vi "VI Tree.vi"   [LabVIEW 2015, in "Keithley 2600 Series.lvlib"]
doc: "This is the instrument driver for the Keithley 2600 Series. The VI Tree displays all the user-callable VIs of the instrument driver in an organized table."
uses:
  Keithley 2600 Series.lvlib
  Configure/Factory Script/Configure Tag Current Pulse (Linear).vi
  Configure/Factory Script/Configure Tag Voltage Pulse (Linear).vi
  Configure/Source/Configure Source (Level).vi
  Data/Read Asynchronous Measurement (Current).vi
  Data/Read Current (Linear Voltage Sweep).vi
  Data/Read Measurement (Current).vi
  Data/Read Transconductance (Current).vi
  Data/Read Voltage (Linear Current Sweep).vi
panel:
  # "(c) 2020 - 2022 National Instruments.  ALL RIGHTS RESERVED."
  # "SEE DIAGRAM\nFOR VI TREE."
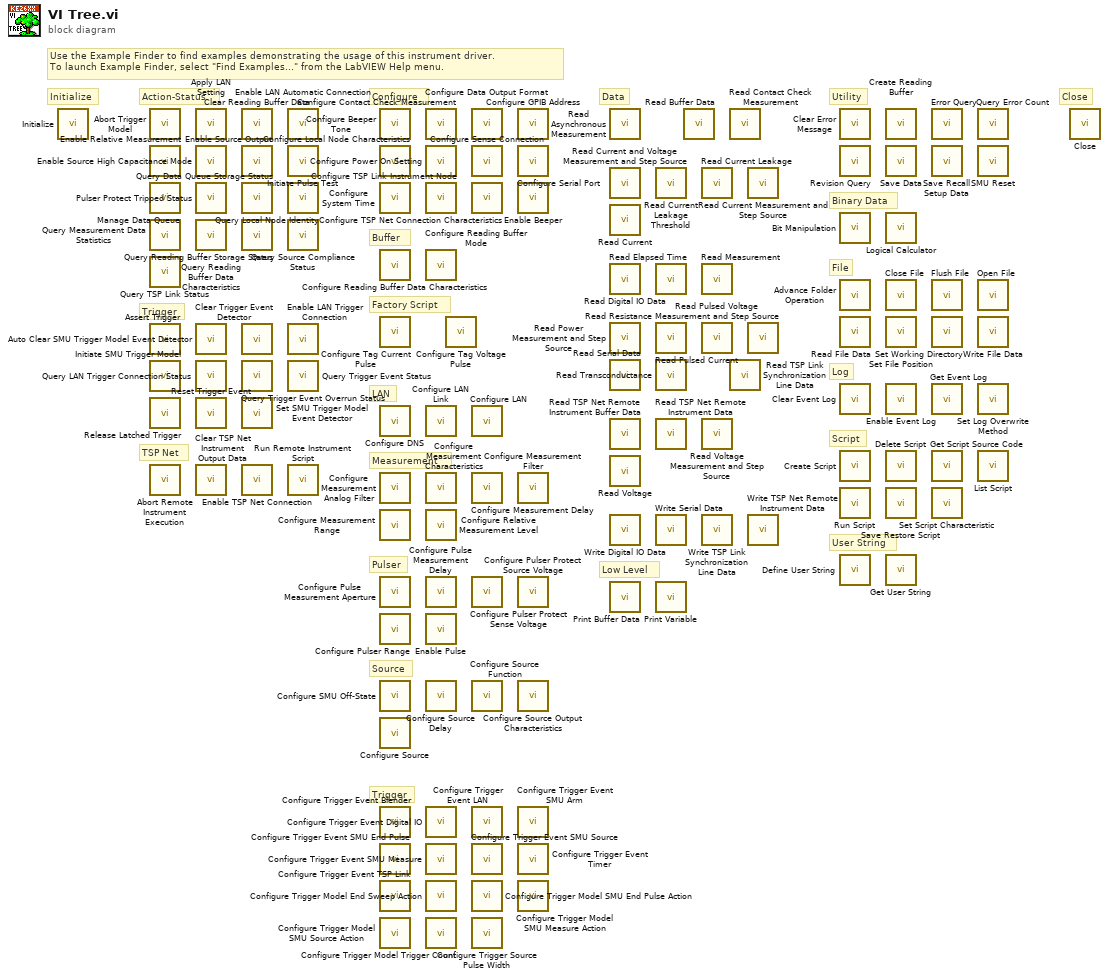
[diagram p0: block diagram]
diagram:
  # "Close"
  # "User String"
  # "Script"
  # "Log"
  # "File"
  # "Binary Data"
  # "Utility"
  # "Low Level"
  # "Data"
  # "Trigger"
  # "Source"
  # "Pulser"
  # "Measurement"
  # "LAN"
  # "Factory Script"
  # "Buffer"
  # "Configure"
  # "TSP Net"
  # "Trigger"
  # "Action-Status"
  # "Initialize"
  # "Use the Example Finder to find examples demonstrating the usage of this instrument driver.\nTo launch Example Finder, select \"Find Examples...\" from the LabVIEW Help menu."
  n1 = call "Initialize.vi"() -> ()  [unwired: 10 in, 2 out]
  n2 = call "Abort Trigger Model.vi"() -> ()  [unwired: 10 in, 2 out]
  n3 = call "Enable Relative Measurement.vi"() -> ()  [unwired: 10 in, 2 out]
  n4 = call "Manage Data Queue.vi"() -> ()  [unwired: 9 in, 3 out]
  n5 = call "Query Measurement Data Statistics.vi"() -> ()  [unwired: 9 in, 3 out]
  n6 = call "Query TSP Link Status.vi"() -> ()  [unwired: 9 in, 3 out]
  n7 = call "Assert Trigger.vi"() -> ()  [unwired: 10 in, 2 out]
  n8 = call "Initiate SMU Trigger Model.vi"() -> ()  [unwired: 10 in, 2 out]
  n9 = call "Release Latched Trigger.vi"() -> ()  [unwired: 10 in, 2 out]
  n10 = call "Abort Remote Instrument Execution.vi"() -> ()  [unwired: 10 in, 2 out]
  n11 = call "Apply LAN Setting.vi"() -> ()  [unwired: 10 in, 2 out]
  n12 = call "Enable Source High Capacitance Mode.vi"() -> ()  [unwired: 10 in, 2 out]
  n13 = call "Pulser Protect Tripped Status.vi"() -> ()  [unwired: 9 in, 3 out]
  n14 = call "Query Reading Buffer Data Characteristics.vi"() -> ()  [unwired: 9 in, 7 out]
  n15 = call "Auto Clear SMU Trigger Model Event Detector.vi"() -> ()  [unwired: 10 in, 2 out]
  n16 = call "Query LAN Trigger Connection Status.vi"() -> ()  [unwired: 9 in, 3 out]
  n17 = call "Reset Trigger Event.vi"() -> ()  [unwired: 10 in, 2 out]
  n18 = call "Clear TSP Net Instrument Output Data.vi"() -> ()  [unwired: 10 in, 2 out]
  n19 = call "Clear Reading Buffer Data.vi"() -> ()  [unwired: 10 in, 2 out]
  n20 = call "Enable Source Output.vi"() -> ()  [unwired: 10 in, 2 out]
  n21 = call "Query Data Queue Storage Status.vi"() -> ()  [unwired: 8 in, 4 out]
  n22 = call "Query Reading Buffer Storage Status.vi"() -> ()  [unwired: 7 in, 5 out]
  n23 = call "Clear Trigger Event Detector.vi"() -> ()  [unwired: 10 in, 2 out]
  n24 = call "Query Trigger Event Overrun Status.vi"() -> ()  [unwired: 9 in, 3 out]
  n25 = call "Set SMU Trigger Model Event Detector.vi"() -> ()  [unwired: 10 in, 2 out]
  n26 = call "Enable TSP Net Connection.vi"() -> ()  [unwired: 14 in, 2 out]
  n27 = call "Enable LAN Automatic Connection.vi"() -> ()  [unwired: 10 in, 2 out]
  n28 = call "Initiate Pulse Test.vi"() -> ()  [unwired: 10 in, 2 out]
  n29 = call "Query Local Node Identity.vi"() -> ()  [unwired: 7 in, 5 out]
  n30 = call "Query Source Compliance Status.vi"() -> ()  [unwired: 9 in, 3 out]
  n31 = call "Enable LAN Trigger Connection.vi"() -> ()  [unwired: 10 in, 2 out]
  n32 = call "Query Trigger Event Status.vi"() -> ()  [unwired: 9 in, 3 out]
  n33 = call "Run Remote Instrument Script.vi"() -> ()  [unwired: 10 in, 2 out]
  n34 = call "Configure Beeper Tone.vi"() -> ()  [unwired: 10 in, 2 out]
  n35 = call "Configure Local Node Characteristics.vi"() -> ()  [unwired: 14 in, 2 out]
  n36 = call "Configure System Time.vi"() -> ()  [unwired: 10 in, 2 out]
  n37 = call "Configure Reading Buffer Data Characteristics.vi"() -> ()  [unwired: 10 in, 2 out]
  n38 = call-poly "Configure Tag Current Pulse.vi"() -> ()  [unwired: 26 in, 2 out]
  n39 = call "Configure DNS.vi"() -> ()  [unwired: 14 in, 2 out]
  n40 = call "Configure Measurement Analog Filter.vi"() -> ()  [unwired: 10 in, 2 out]
  n41 = call "Configure Measurement Range.vi"() -> ()  [unwired: 14 in, 2 out]
  n42 = call "Configure Pulse Measurement Aperture.vi"() -> ()  [unwired: 10 in, 2 out]
  n43 = call "Configure Pulser Range.vi"() -> ()  [unwired: 10 in, 2 out]
  n44 = call "Configure SMU Off-State.vi"() -> ()  [unwired: 10 in, 2 out]
  n45 = call-poly "Configure Source.vi"() -> ()  [unwired: 14 in, 2 out]
  n46 = call "Configure Trigger Event Blender.vi"() -> ()  [unwired: 14 in, 2 out]
  n47 = call "Configure Trigger Event SMU End Pulse.vi"() -> ()  [unwired: 14 in, 2 out]
  n48 = call "Configure Trigger Event TSP Link.vi"() -> ()  [unwired: 14 in, 2 out]
  n49 = call "Configure Trigger Model SMU Source Action.vi"() -> ()  [unwired: 18 in, 2 out]
  n50 = call "Configure Contact Check Measurement.vi"() -> ()  [unwired: 10 in, 2 out]
  n51 = call "Configure Power On Setting.vi"() -> ()  [unwired: 10 in, 2 out]
  n52 = call "Configure TSP Link Instrument Node.vi"() -> ()  [unwired: 10 in, 2 out]
  n53 = call "Configure Reading Buffer Mode.vi"() -> ()  [unwired: 14 in, 2 out]
  n54 = call "Configure LAN Link.vi"() -> ()  [unwired: 14 in, 2 out]
  n55 = call "Configure Measurement Characteristics.vi"() -> ()  [unwired: 10 in, 2 out]
  n56 = call "Configure Relative Measurement Level.vi"() -> ()  [unwired: 14 in, 2 out]
  n57 = call "Configure Pulse Measurement Delay.vi"() -> ()  [unwired: 10 in, 2 out]
  n58 = call "Enable Pulse.vi"() -> ()  [unwired: 10 in, 2 out]
  n59 = call "Configure Source Delay.vi"() -> ()  [unwired: 10 in, 2 out]
  n60 = call "Configure Trigger Event Digital IO.vi"() -> ()  [unwired: 14 in, 2 out]
  n61 = call "Configure Trigger Event SMU Measure.vi"() -> ()  [unwired: 14 in, 2 out]
  n62 = call "Configure Trigger Model End Sweep Action.vi"() -> ()  [unwired: 10 in, 2 out]
  n63 = call "Configure Trigger Model Trigger Count.vi"() -> ()  [unwired: 10 in, 2 out]
  n64 = call-poly "Configure Tag Voltage Pulse.vi"() -> ()  [unwired: 26 in, 2 out]
  n65 = call "Configure Data Output Format.vi"() -> ()  [unwired: 10 in, 2 out]
  n66 = call "Configure Sense Connection.vi"() -> ()  [unwired: 10 in, 2 out]
  n67 = call "Configure TSP Net Connection Characteristics.vi"() -> ()  [unwired: 10 in, 2 out]
  n68 = call "Configure LAN.vi"() -> ()  [unwired: 10 in, 2 out]
  n69 = call "Configure Measurement Delay.vi"() -> ()  [unwired: 10 in, 2 out]
  n70 = call "Configure Pulser Protect Sense Voltage.vi"() -> ()  [unwired: 10 in, 2 out]
  n71 = call "Configure Source Function.vi"() -> ()  [unwired: 10 in, 2 out]
  n72 = call "Configure Trigger Event LAN.vi"() -> ()  [unwired: 14 in, 2 out]
  n73 = call "Configure Trigger Event SMU Source.vi"() -> ()  [unwired: 14 in, 2 out]
  n74 = call "Configure Trigger Model SMU End Pulse Action.vi"() -> ()  [unwired: 14 in, 2 out]
  n75 = call "Configure Trigger Source Pulse Width.vi"() -> ()  [unwired: 14 in, 2 out]
  n76 = call "Configure GPIB Address.vi"() -> ()  [unwired: 10 in, 2 out]
  n77 = call "Configure Serial Port.vi"() -> ()  [unwired: 10 in, 2 out]
  n78 = call "Enable Beeper.vi"() -> ()  [unwired: 10 in, 2 out]
  n79 = call "Configure Measurement Filter.vi"() -> ()  [unwired: 10 in, 2 out]
  n80 = call "Configure Pulser Protect Source Voltage.vi"() -> ()  [unwired: 10 in, 2 out]
  n81 = call "Configure Source Output Characteristics.vi"() -> ()  [unwired: 10 in, 2 out]
  n82 = call "Configure Trigger Event SMU Arm.vi"() -> ()  [unwired: 14 in, 2 out]
  n83 = call "Configure Trigger Event Timer.vi"() -> ()  [unwired: 14 in, 2 out]
  n84 = call "Configure Trigger Model SMU Measure Action.vi"() -> ()  [unwired: 14 in, 2 out]
  n85 = call-poly "Read Asynchronous Measurement.vi"() -> ()  [unwired: 9 in, 3 out]
  n86 = call "Read Current and Voltage Measurement and Step Source.vi"() -> ()  [unwired: 8 in, 4 out]
  n87 = call-poly "Read Current.vi"() -> ()  [unwired: 9 in, 3 out]
  n88 = call "Read Digital IO Data.vi"() -> ()  [unwired: 8 in, 4 out]
  n89 = call "Read Power Measurement and Step Source.vi"() -> ()  [unwired: 9 in, 3 out]
  n90 = call "Read Serial Data.vi"() -> ()  [unwired: 9 in, 3 out]
  n91 = call "Read TSP Net Remote Instrument Buffer Data.vi"() -> ()  [unwired: 9 in, 3 out]
  n92 = call-poly "Read Voltage.vi"() -> ()  [unwired: 9 in, 3 out]
  n93 = call "Write Digital IO Data.vi"() -> ()  [unwired: 10 in, 2 out]
  n94 = call "Print Buffer Data.vi"() -> ()  [unwired: 9 in, 3 out]
  n95 = call "Read Current Leakage Threshold.vi"() -> ()  [unwired: 13 in, 3 out]
  n96 = call "Read Elapsed Time.vi"() -> ()  [unwired: 9 in, 3 out]
  n97 = call "Read Pulsed Current.vi"() -> ()  [unwired: 13 in, 3 out]
  n98 = call-poly "Read Transconductance.vi"() -> ()  [unwired: 11 in, 5 out]
  n99 = call "Read TSP Net Remote Instrument Data.vi"() -> ()  [unwired: 9 in, 3 out]
  n100 = call "Write Serial Data.vi"() -> ()  [unwired: 10 in, 2 out]
  n101 = call "Print Variable.vi"() -> ()  [unwired: 8 in, 4 out]
  n102 = call "Read Buffer Data.vi"() -> ()  [unwired: 7 in, 5 out]
  n103 = call "Read Current Leakage.vi"() -> ()  [unwired: 13 in, 3 out]
  n104 = call-poly "Read Measurement.vi"() -> ()  [unwired: 8 in, 4 out]
  n105 = call "Read Pulsed Voltage.vi"() -> ()  [unwired: 13 in, 3 out]
  n106 = call "Read Voltage Measurement and Step Source.vi"() -> ()  [unwired: 9 in, 3 out]
  n107 = call "Write TSP Link Synchronization Line Data.vi"() -> ()  [unwired: 10 in, 2 out]
  n108 = call "Read Contact Check Measurement.vi"() -> ()  [unwired: 7 in, 5 out]
  n109 = call "Read TSP Link Synchronization Line Data.vi"() -> ()  [unwired: 8 in, 4 out]
  n110 = call "Read Current Measurement and Step Source.vi"() -> ()  [unwired: 9 in, 3 out]
  n111 = call "Read Resistance Measurement and Step Source.vi"() -> ()  [unwired: 9 in, 3 out]
  n112 = call "Write TSP Net Remote Instrument Data.vi"() -> ()  [unwired: 10 in, 2 out]
  n113 = call "Clear Error Message.vi"() -> ()  [unwired: 10 in, 2 out]
  n114 = call "Revision Query.vi"() -> ()  [unwired: 8 in, 4 out]
  n115 = call "Bit Manipulation.vi"() -> ()  [unwired: 9 in, 3 out]
  n116 = call "Advance Folder Operation.vi"() -> ()  [unwired: 10 in, 6 out]
  n117 = call "Read File Data.vi"() -> ()  [unwired: 9 in, 3 out]
  n118 = call "Clear Event Log.vi"() -> ()  [unwired: 10 in, 2 out]
  n119 = call "Create Script.vi"() -> ()  [unwired: 10 in, 2 out]
  n120 = call "Run Script.vi"() -> ()  [unwired: 10 in, 2 out]
  n121 = call "Define User String.vi"() -> ()  [unwired: 10 in, 2 out]
  n122 = call "Create Reading Buffer.vi"() -> ()  [unwired: 10 in, 2 out]
  n123 = call "Save Data.vi"() -> ()  [unwired: 14 in, 2 out]
  n124 = call "Logical Calculator.vi"() -> ()  [unwired: 9 in, 3 out]
  n125 = call "Close File.vi"() -> ()  [unwired: 10 in, 2 out]
  n126 = call "Set File Position.vi"() -> ()  [unwired: 8 in, 4 out]
  n127 = call "Enable Event Log.vi"() -> ()  [unwired: 10 in, 2 out]
  n128 = call "Delete Script.vi"() -> ()  [unwired: 10 in, 2 out]
  n129 = call "Save Restore Script.vi"() -> ()  [unwired: 10 in, 2 out]
  n130 = call "Get User String.vi"() -> ()  [unwired: 9 in, 3 out]
  n131 = call "Error Query.vi"() -> ()  [unwired: 8 in, 4 out]
  n132 = call "Save Recall Setup Data.vi"() -> ()  [unwired: 10 in, 2 out]
  n133 = call "Flush File.vi"() -> ()  [unwired: 10 in, 2 out]
  n134 = call "Set Working Directory.vi"() -> ()  [unwired: 9 in, 3 out]
  n135 = call "Get Event Log.vi"() -> ()  [unwired: 8 in, 4 out]
  n136 = call "Get Script Source Code.vi"() -> ()  [unwired: 9 in, 3 out]
  n137 = call "Set Script Characteristic.vi"() -> ()  [unwired: 10 in, 2 out]
  n138 = call "Query Error Count.vi"() -> ()  [unwired: 9 in, 3 out]
  n139 = call "SMU Reset.vi"() -> ()  [unwired: 10 in, 2 out]
  n140 = call "Open File.vi"() -> ()  [unwired: 10 in, 2 out]
  n141 = call "Write File Data.vi"() -> ()  [unwired: 10 in, 2 out]
  n142 = call "Set Log Overwrite Method.vi"() -> ()  [unwired: 10 in, 2 out]
  n143 = call "List Script.vi"() -> ()  [unwired: 9 in, 3 out]
  n144 = call "Close.vi"() -> ()  [unwired: 11 in, 1 out]
